vi "EV Util - Get single memory list value.vi"(1 "Memory list value name":string) -> (0 "Output single value":dbl)   [LabVIEW 2016]
uses:
  custom and Sc run Seq Sub VIs (x64).llb/memlist data type.ctl
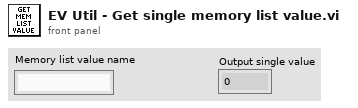
[diagram p1: front panel]
types:
  T1 = typedef "memlist data type.ctl" = enum32{"curve", "value", "result", "waveform"}
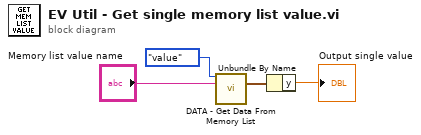
[diagram p0: block diagram]
diagram:
  n1 = call "DATA - Get Data From Memory List.vi"("Data type"=memlist_data_type."value", "Data Name"="Memory list value name") -> ("value"=w2:cluster{"x":dbl, "y":dbl, "z":dbl})  [unwired: 7 in, 6 out]
  n2 = Unbundle By Name(w2) -> ("y"=→"Output single value":dbl)
